vi "ErrCheck_SettingsVariablesPresent.vi"(8 "error in (no error)":errorcluster, 10 "Settings Array IN":T1[](array[typedef]), 11 "Settings type string":string) -> (0 "error out":errorcluster, 2 "Error String":string, 3 "Error?":bool)   [LabVIEW 2012]
doc: "SciScan 1.2 160622"
uses:
  MacroGUI Module/Custom Controls and Typedefs/GFG Variable for IO.ctl
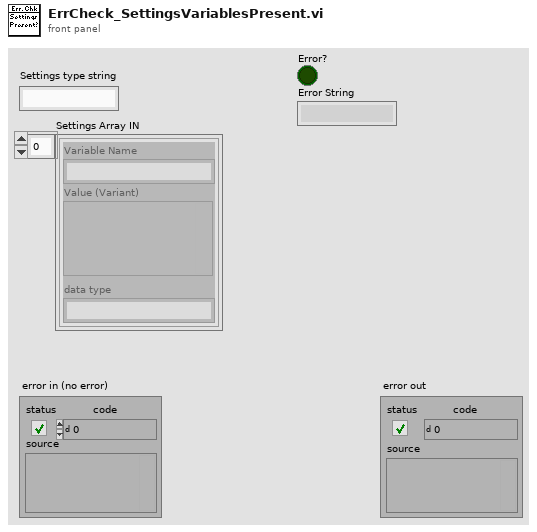
[diagram p1: front panel]
types:
  T1 = typedef "GFG Variable for IO.ctl" = cluster{"Variable Name":string, "Value (Variant)":variant, "data type":string}
  T2 = enum16{"Get Settings Table ", "Read Settings File", "Get Specified Settings"}
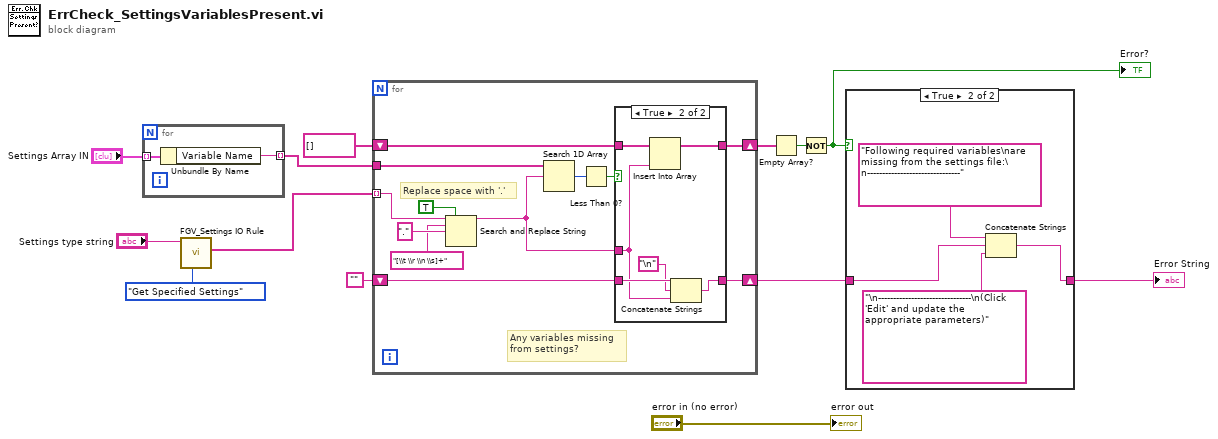
[diagram p0: block diagram]
diagram:
  n1 = for {
    tunnel: "Settings Array IN" -> [w15] mode=indexing
    tunnel: [w14] -> w9 mode=indexing
    n2 = Unbundle By Name(w15) -> ("Variable Name"=w14:string)
  }
  n3 = call "FGV_Settings IO Rule.vi"("Command_Settings IO Rule"=T2."Get Specified Settings", "Settings Type IN"="Settings type string") -> ("Specified Settings (OUT)"=w11:string[])  [unwired: 7 in, 2 out]
  n4 = for {
    tunnel: w11 -> [w18] mode=indexing
    tunnel: w9 -> [w27]
    shift-right: [w23] -> w7
    shift-left: string[] [] ("Specified Settings (OUT)") -> [w24]
    shift-right: [w21] -> w3
    shift-left: "" -> [w22]
    # "Replace space with '.'"
    # "Any variables missing from settings?"
    n5 = Search and Replace String(replace all?=TRUE ("replace all? (F)"), input string=w18, search string="[\\t \\r \\n \\s]+", replace string="." ("replace string (\"\")")) -> (result string=w17:string)  [unwired: 4 in, 3 out]
    n6 = Search 1D Array(1D array=w27, element=w17) -> (index of element=w26:i32)  [unwired: 1 in]
    n7 = Less Than 0?(x=w26) -> (x < 0?=w25:bool)
    n8 = case shown="True" w25 {
      tunnel: w24 -> [w28 w35]
      tunnel: w17 -> [_ w31]
      tunnel: [w28 w34] -> w23
      tunnel: w22 -> [w29 w33]
      tunnel: [w29 w30] -> w21
      frame False {
      }
      frame True {
        n9 = Insert Into Array(array=w35, new element=w31) -> (w34:string[])  [unwired: 1 in]
        n10 = Concatenate Strings(w33, "\n", w31) -> (w30:string)
      }
    }
  }
  n11 = Empty Array?(array=w7) -> (empty?=w6:bool)
  n12 = Not(x=w6) -> (.not. x?=w5:bool)
  "Error?" <- w5
  n13 = case shown="True" w5 {
    tunnel: w3 -> [_ w38]
    tunnel: [_ w37] -> w2
    frame False {
    }
    frame True {
      n14 = Concatenate Strings("Following required variables\nare missing from the settings file:\n-------------------------------", w38, "\n-------------------------------\n(Click 'Edit' and update the appropriate parameters)" ("string")) -> (w37:string)
    }
  }
  "Error String" <- w2
  "error out" <- "error in (no error)"
